vi "test.vi"() -> ()   [LabVIEW 2013]
panel:
  out "Boolean":bool
  in  "x":dbl
  # "test change change change is comingggg"
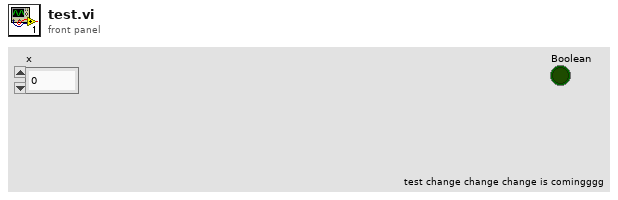
[diagram p1: front panel]
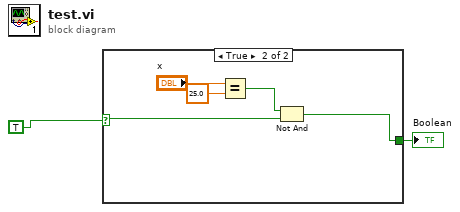
[diagram p0: block diagram]
diagram:
  n1 = case shown="True" TRUE {
    selector: TRUE -> [w3 w8]
    tunnel: [w3 w4] -> w1
    frame False {
    }
    frame True {
      n2 = Equal?(x="x", y=25.0) -> (x = y?=w7:bool)
      n3 = Not And(1:w8, 2:w7) -> (0:w4:bool)
    }
  }
  "Boolean" <- w1
